vi "Frame&Parity Cancel.vi"(8 "error in (no error)":errorcluster, 11 "Error Cancellation (Def:On)":bool) -> (0 "error out":errorcluster)   [LabVIEW 2019]
uses:
  <vilib>/Utility/error.llb/DialogType.ctl
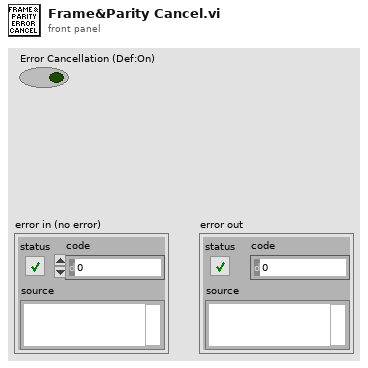
[diagram p1: front panel]
types:
  T1 = typedef "DialogType.ctl" = u16
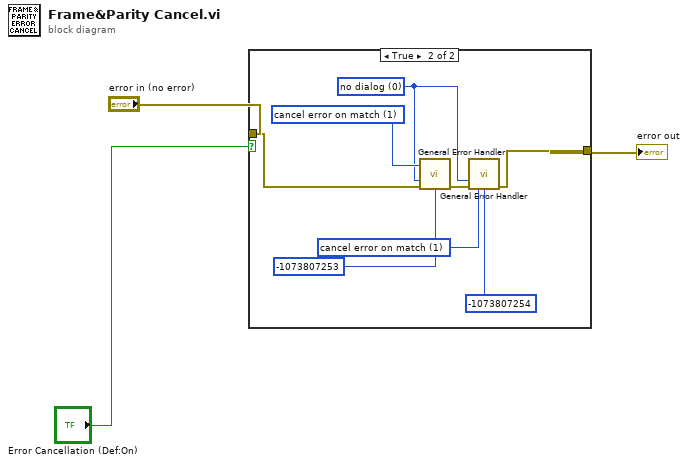
[diagram p0: block diagram]
diagram:
  n1 = case shown="True" "Error Cancellation (Def:On)" {
    tunnel: "error in (no error)" -> [w4 w5]
    tunnel: [w4 w10] -> w1
    frame False {
    }
    frame True {
      w6 = T1 0 items=["no dialog", "OK message", "continue or stop message", "OK message + warnings", "continue/stop + warnings"] ("type of dialog (OK msg:1)")
      w7 = 1 items=["no exception", "cancel error on match", "set error on match"] ("[exception action] (none:0)")
      w9 = 1 items=["no exception", "cancel error on match", "set error on match"] ("[exception action] (none:0)")
      n2 = call <vilib>:"General Error Handler.vi"("type of dialog (OK msg:1)"=w6, "error in (no error)"=w5, "[exception action] (none:0)"=w9, "[exception code]"=-1073807253) -> ("error out"=w11:errorcluster)  [unwired: 7 in, 4 out]
      n3 = call <vilib>:"General Error Handler.vi"("type of dialog (OK msg:1)"=w6, "error in (no error)"=w11, "[exception action] (none:0)"=w7, "[exception code]"=-1073807254 ("[exception code] 2")) -> ("error out"=w10:errorcluster)  [unwired: 7 in, 4 out]
    }
  }
  "error out" <- w1
